vi "Get Window DPI.vi"(8 "error in":errorcluster caption="error in (no error)" {"code" format="%d\n%x"}, 11 "window refnum in":T1 caption="window refnum in (NaWR)") -> (0 "error out":errorcluster {"code" format="%d\n%x"}, 2 "DPI":i32, 3 "window refnum out":T1)   [LabVIEW 2020, in "MacroAssert.lvlib" / "Win Util.lvlib"]
doc: "This VI will use window refnum in to get the name of a window. The name of a window is simply the text appearing in the title bar of the window. If the title bar of the window is not shown, the name of the window will be a NULL string."
uses:
  Win Util.lvlib
  user32.dll
  SHCore.dll
  Window Refnum.ctl
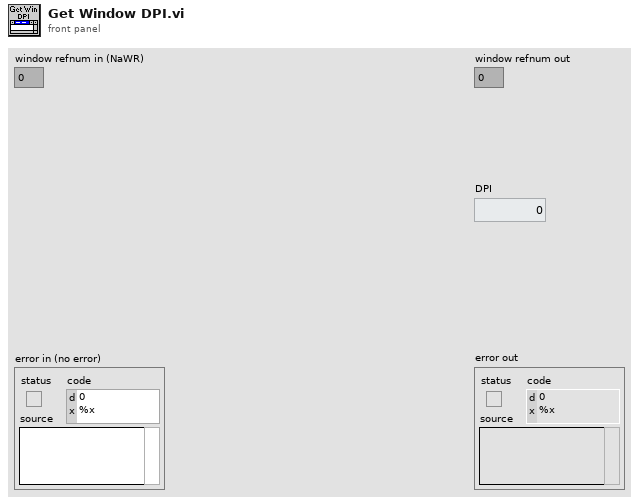
[diagram p1: front panel]
types:
  T1 = typedef "MacroAssert.lvlib/Win Util.lvlib/Window Refnum.ctl" = u64
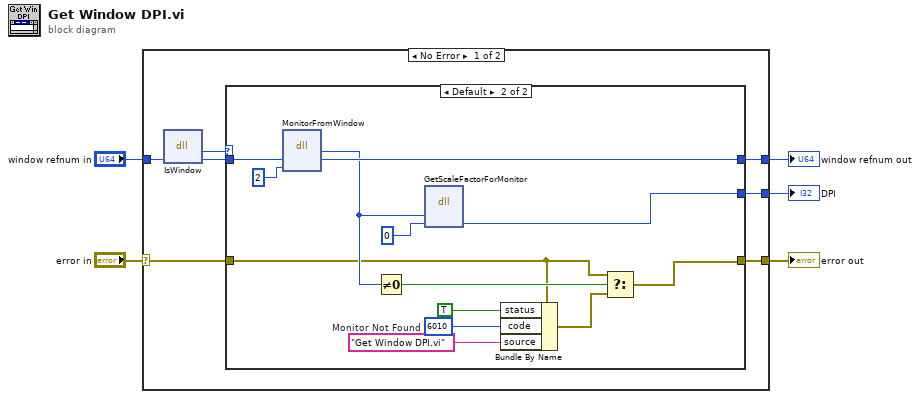
[diagram p0: block diagram]
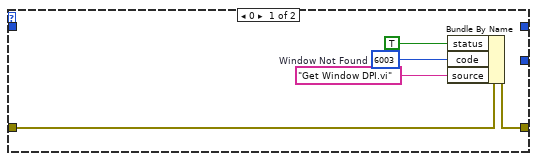
[diagram p2: hidden frame]
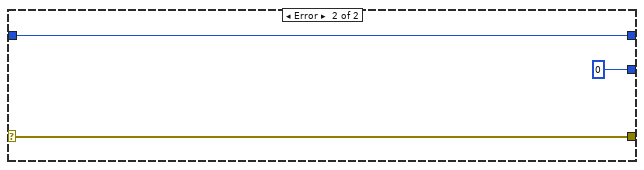
[diagram p3: hidden frame]
diagram:
  n1 = case shown="No Error" "error in" {
    selector: "error in" -> [w11 w33]
    tunnel: "window refnum in" -> [w12 w32]
    tunnel: [w10 w33] -> w4
    tunnel: [w7 0] -> w2
    tunnel: [w6 w32] -> w3
    frame No Error {
      n2 = dll-call lib="user32.dll" fn="IsWindow"("hWnd"=w12) -> ("IsWindow?"=w9:i32, "hWnd"=w8:u64)  [unwired: 3 in, 2 out]
      n3 = case shown="Default" w9 {
        tunnel: w11 -> [w14 w18]
        tunnel: [w17 w20] -> w10
        tunnel: w8 -> [_ w28]
        tunnel: [_ w27] -> w7
        tunnel: [_ w26] -> w6
        frame 0 {
          w16 = 6003  # Window Not Found
          n4 = Bundle By Name(cluster=w14, "status"=TRUE ("show call chain? (False)"), "code"=w16, "source"="Get Window DPI.vi") -> (w17:errorcluster)
        }
        frame Default {
          w22 = 6010  # Monitor Not Found
          n5 = dll-call lib="USER32.DLL" fn="MonitorFromWindow"("hWnd"=w28, "dwFlags"=u32 2) -> ("Return Value"=w25:u32, "hWnd"=w26:u64)  [unwired: 4 in, 2 out]
          n6 = Not Equal To 0?(x=w25) -> (x != 0?=w24:bool)
          n7 = dll-call lib="SHCore.dll" fn="GetScaleFactorForMonitor"("hMon"=w25, "pScale"=0) -> ("pScale"=w27:i32)  [unwired: 4 in, 3 out]
          n8 = Bundle By Name(cluster=w18, "status"=TRUE ("show call chain? (False)"), "code"=w22, "source"="Get Window DPI.vi") -> (w19:errorcluster)
          n9 = Select(t=w18, s=w24, f=w19) -> (s? t:f=w20:errorcluster)
        }
      }
    }
    frame Error {
    }
  }
  "error out" <- w4
  "window refnum out" <- w3
  "DPI" <- w2
